vi "Check DAQ Registry Empty.vi"(8 "error in (no error)":errorcluster, 11 "FP Controls in":refnum<class "FP Controls.lvclass">) -> (0 "error out":errorcluster, 2 "DAQ Reg Empty?":bool, 3 "FP Controls out":refnum<class "FP Controls.lvclass">)   [LabVIEW 2018, in "Configuration Grandmaster.lvlib" / "FP Controls.lvclass"]
uses:
  FP Controls.lvclass
  FP Controls.lvclass/FP Controls.ctl
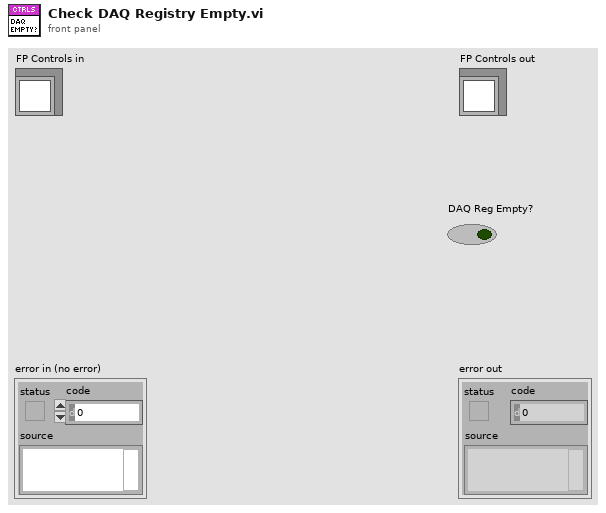
[diagram p1: front panel]
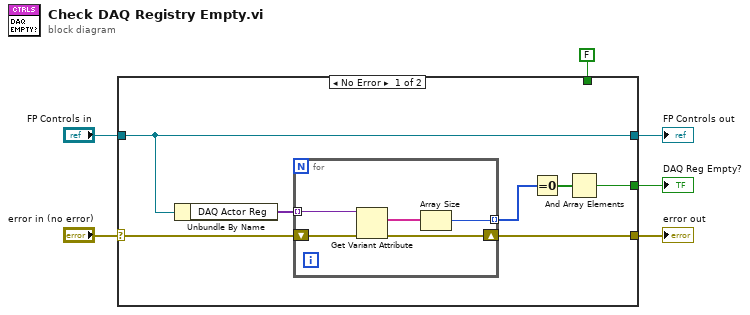
[diagram p0: block diagram]
diagram:
  n1 = case shown="No Error" "error in (no error)" {
    selector: "error in (no error)" -> [w11 w21]
    tunnel: [w10 w21] -> w5
    tunnel: [w13 w20] -> w3
    tunnel: "FP Controls in" -> [w13 w20]
    tunnel: [w7 w19] -> w2
    tunnel: FALSE -> [_ w19]
    frame No Error {
      n2 = Unbundle By Name(w13) -> ("DAQ Actor Reg"=w12:variant[])
      n3 = for {
        tunnel: w12 -> [w18] mode=indexing
        tunnel: [w16] -> w9 mode=indexing
        shift-right: [w14] -> w10
        shift-left: w11 -> [w15]
        n4 = Get Variant Attribute(Variant=w18, error in=w15) -> (names=w17:string[], error out=w14:errorcluster)  [unwired: 2 in, 2 out]
        n5 = Array Size(array=w17) -> (size(s)=w16:i32)
      }
      n6 = Equal To 0?(x=w9) -> (x = 0?=w8:bool[])
      n7 = And Array Elements(Boolean array=w8) -> (logical AND=w7:bool)
    }
    frame Error {
    }
  }
  "error out" <- w5
  "FP Controls out" <- w3
  "DAQ Reg Empty?" <- w2
